vi "Calculate F(x) - Optimized (1).vi"() -> (3 "Output Array":dbl[][](array[numeric]), 4 "val1":dbl, 6 "f(x)":dbl, 8 "x-y":dbl, 14 "Waveform Graph":dbl[](graph), 15 "Waveform Graph 2":dbl[](graph))   [LabVIEW 2021]
doc: "This is the optimized Calculate F(x) which will take only 250ms to 320ms to execute, whereas the previous version will take atleast 10 min to execute."
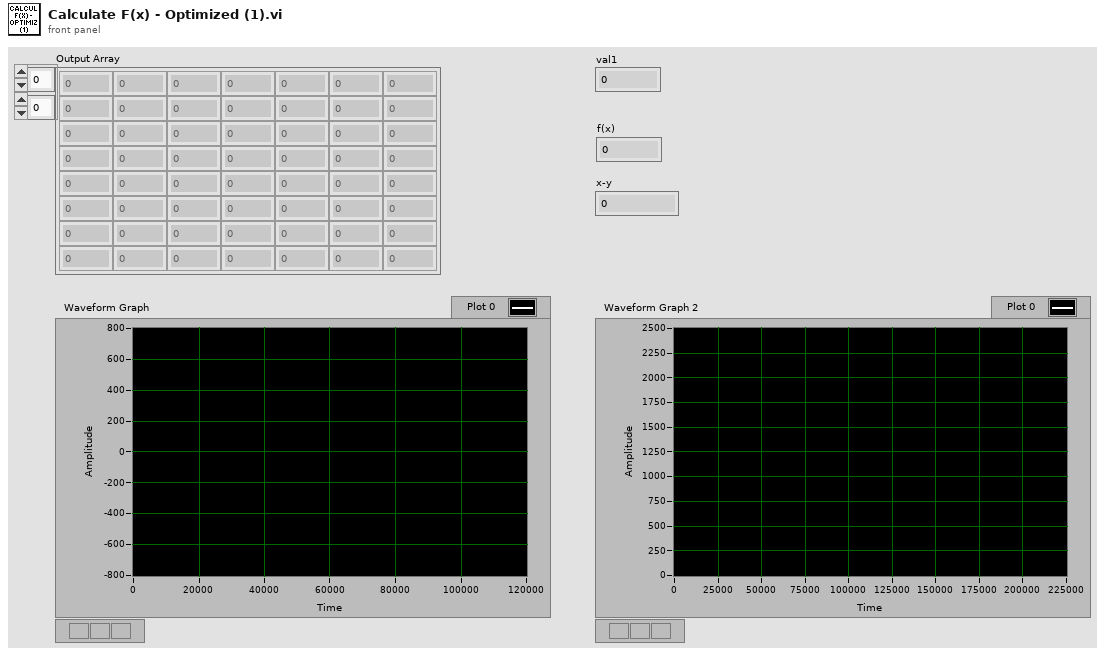
[diagram p1: front panel]
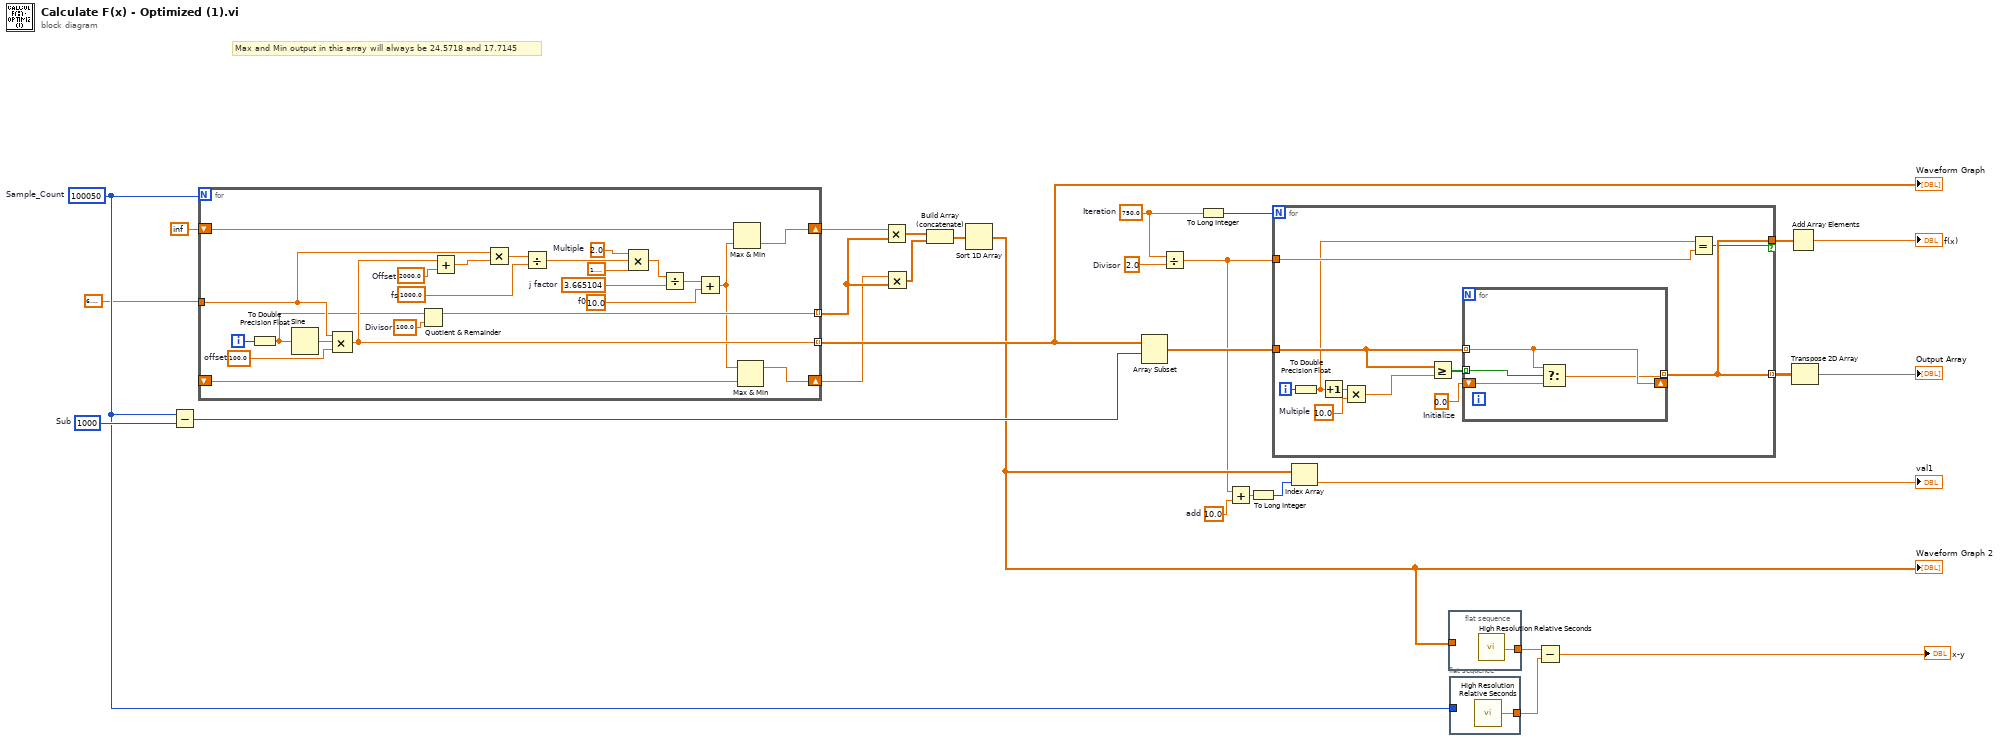
[diagram p0: block diagram]
diagram:
  w3 = 750.0  # Iteration
  w17 = 100050  # Sample_Count
  w25 = 1000  # Sub
  w27 = 10.0  # add
  w29 = 2.0  # Divisor
  # "Max and Min output in this array will always be 24.5718 and 17.7145"
  n1 = Subtract(x=w17, y=w25) -> (x-y=w23:i32)
  n2 = for {
    N: w17 -> [_]
    tunnel: 6.283185307179586 -> [w42]
    tunnel: [w43] -> w22 mode=indexing
    shift-right: [w39] -> w13
    shift-left: inf -> [w40]
    shift-right: [w38] -> w12
    shift-left: _ -> [w41]
    tunnel: [w37] -> w16 mode=indexing
    i -> [w35]
    w31 = 2.0  # Multiple
    w47 = 10.0  # f0
    w46 = 3.665104  # j factor
    w44 = 1000.0  # fs
    w45 = 2000.0  # Offset
    w51 = 100.0  # Divisor
    w52 = 100.0  # offset
    n3 = To Double Precision Float(number=w35) -> (double precision float=w34:dbl)
    n4 = Sine(x=w34) -> (sin(x)=w53:dbl)
    n5 = Compound Arithmetic op=MULTIPLY(w42, w53, w52) -> (w43:dbl)
    n6 = Quotient & Remainder(x=w34, y=w51) -> (x-y*floor(x/y)=w37:dbl)  [unwired: 1 out]
    n7 = Add(x=w43, y=w45) -> (x+y=w49:dbl)
    n8 = Multiply(x=w42, y=w49) -> (x*y=w48:dbl)
    n9 = Divide(x=w48, y=w44) -> (x/y=w32:dbl)
    n10 = Compound Arithmetic op=MULTIPLY(w31, w32, 1.5707963267948966) -> (w33:dbl)
    n11 = Divide(x=w33, y=w46) -> (x/y=w50:dbl)
    n12 = Add(x=w50, y=w47) -> (x+y=w36:dbl)
    n13 = Max & Min(x=w40, y=w36) -> (min(x,y)=w39:dbl)  [unwired: 1 out]
    n14 = Max & Min(x=w36, y=w41) -> (max(x,y)=w38:dbl)  [unwired: 1 out]
  }
  "Waveform Graph" <- w22
  n15 = Multiply(x=w13, y=w16) -> (x*y=w15:dbl[])
  n16 = Multiply(x=w12, y=w16) -> (x*y=w11:dbl[])
  n17 = Build Array (concatenate)(w15, w11) -> (w14:dbl[])
  n18 = Sort 1D Array(array=w14) -> (sorted array=w9:dbl[])
  "Waveform Graph 2" <- w9
  n19 = Array Subset(array=w22, index=w23) -> (w24:dbl[])  [unwired: 1 in]
  n20 = Divide(x=w3, y=w29) -> (x/y=w4:dbl)
  n21 = To Long Integer(number=w3) -> (32bit integer=w2:i32)
  n22 = Add(x=w4, y=w27) -> (x+y=w26:dbl)
  n23 = To Long Integer(number=w26) -> (32bit integer=w1:i32)
  n24 = for {
    N: w2 -> [_]
    tunnel: [w56] -> w8 mode=indexing
    tunnel: w24 -> [w61]
    tunnel: w4 -> [w60]
    tunnel: [w56] -> w6 if=w55
    i -> [w59]
    w57 = 0.0  # Initialize
    w64 = 10.0  # Multiple
    n25 = To Double Precision Float(number=w59) -> (double precision float=w54:dbl)
    n26 = Increment(x=w54) -> (x+1=w63:dbl)
    n27 = Multiply(x=w63, y=w64) -> (x*y=w58:dbl)
    n28 = Greater Or Equal?(x=w61, y=w58) -> (x >= y?=w62:bool[])
    n29 = for {
      tunnel: w61 -> [w67] mode=indexing
      tunnel: w62 -> [w68] mode=indexing
      shift-right: [w67] -> _
      shift-left: w57 -> [w66]
      tunnel: [w65] -> w56 mode=indexing
      n30 = Select(t=w67, s=w68, f=w66) -> (s? t:f=w65:dbl)
    }
    n31 = Equal?(x=w54, y=w60) -> (x = y?=w55:bool)
  }
  n32 = Index Array(array=w9, index=w1) -> (element=→"val1":dbl)
  n33 = flat-sequence {
    tunnel: w9 -> [_]
    tunnel: [w69] -> w20
    frame #0 {
      n34 = call <vilib>:"High Resolution Relative Seconds.vi"() -> ("relative seconds"=w69:dbl)
    }
  }
  n35 = flat-sequence {
    tunnel: w17 -> [_]
    tunnel: [w70] -> w19
    frame #0 {
      n36 = call <vilib>:"High Resolution Relative Seconds.vi"() -> ("relative seconds"=w70:dbl)
    }
  }
  n37 = Subtract(x=w20, y=w19) -> (x-y=→"x-y":dbl)
  n38 = Add Array Elements(numeric array=w6) -> (sum=→"f(x)":dbl)
  n39 = Transpose 2D Array(2D array=w8) -> (transposed array=→"Output Array":dbl[][])
